vi "build token URI.vi"(8 "error in (no error)":errorcluster, 11 "Oauth2 in":refnum<class "Oauth2.lvclass">) -> (0 "error out":errorcluster, 1 "Headers":cluster{"header":string, "value":string}[](array[cluster]), 2 "Token Request URI":string, 3 "Oauth2":refnum<class "Oauth2.lvclass">)   [LabVIEW 2017, in "Oauth2.lvclass"]
uses:
  Oauth2.lvclass
  OAuthToken/OAuth2 Token Element -- enum.ctl
  Oauth2.lvclass/Oauth2.ctl
  <vilib>/LabVIEW Open Source Project/OpenURI/uri/URI.lvclass
  OAuthToken/OAuthAccessToken.lvclass
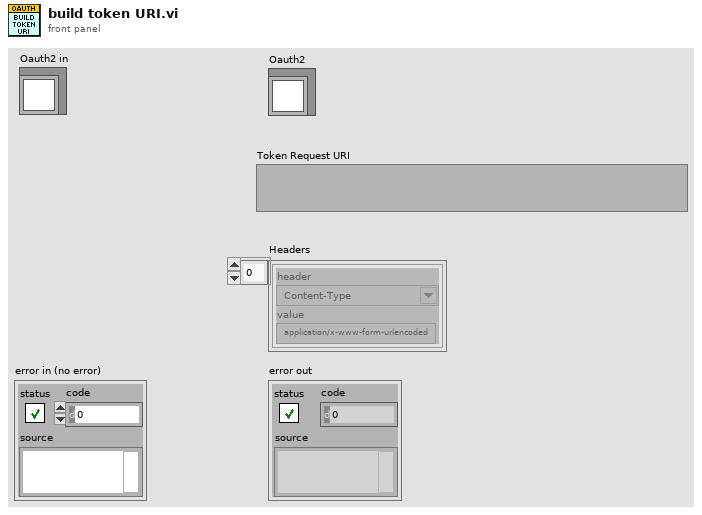
[diagram p1: front panel]
types:
  T1 = typedef "OAuthAccessToken.lvclass/OAuth2 Token Element -- enum.ctl" = enum16{"client_id", "client_secret", "response_type", "scope", "redirect_uri", "error", "error_description", "error_uri", "grant_type", "code", "access_token", "token_type", "expires_in", "username", "password", "refresh_token", "code_challenge", "code_challenge_method", "reverse_proxy_uri", "endpoint element", "access_type", "prompt", "id_token"}
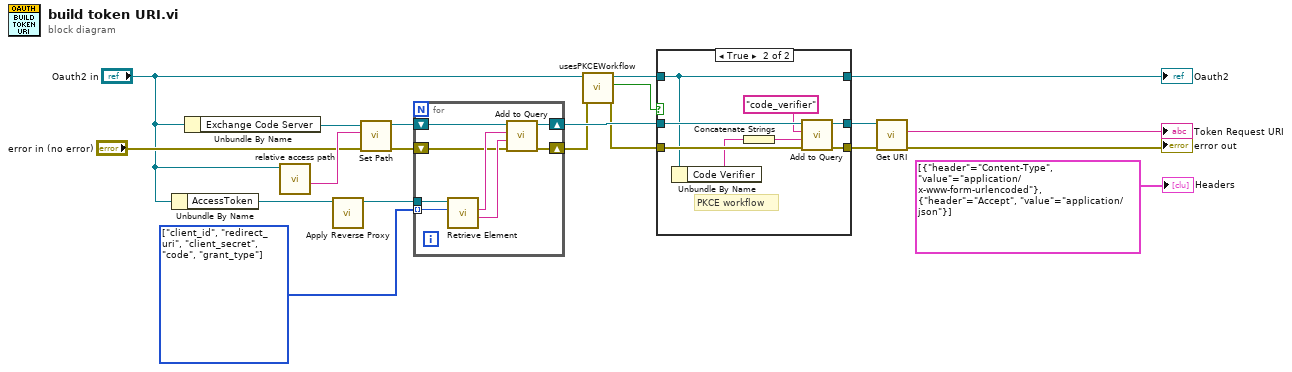
[diagram p0: block diagram]
diagram:
  w15 = T1[] [enum."client_id", enum."redirect_uri", enum."client_secret", enum."code", enum."grant_type"] items=["client_id", "client_secret", "response_type", "scope", "redirect_uri", "error", "error_description", "error_uri", "grant_type", "code", "access_token", "token_type", "expires_in", "username", "password", "refresh_token", "code_challenge", "code_challenge_method", "reverse_proxy_uri", "endpoint element", "access_type", "prompt", "id_token"]
  n1 = Unbundle By Name("Oauth2 in") -> ("AccessToken"=w3:refnum<class "OAuthAccessToken.lvclass">)
  n2 = Unbundle By Name("Oauth2 in") -> ("Exchange Code Server"=w17:refnum<class "URI.lvclass">)
  n3 = call-dynamic "relative access path.vi"("Oauth2 in"="Oauth2 in") -> ("Token Access Path"=w18:string)  [unwired: 9 in, 1 out]
  n4 = call "Apply Reverse Proxy.vi"("OAuthAccessToken in"=w3) -> ("OAuthAccessToken out"=w2:refnum<class "OAuthAccessToken.lvclass">)  [unwired: 9 in, 1 out]
  n5 = call <vilib>:"Set Path.vi"("error in (no error)"="error in (no error)", "path"=w18, "URI in"=w17) -> ("error out"=w13:errorcluster, "URI out"=w14:refnum<class "URI.lvclass">)  [unwired: 7 in]
  n6 = for {
    tunnel: w2 -> [w28]
    tunnel: w15 -> [w27] mode=indexing
    shift-right: [w25] -> w12
    shift-left: w14 -> [w26]
    shift-right: [w21] -> w8
    shift-left: w13 -> [w22]
    n7 = call "Retrieve Element.vi"("Token element"=w27, "OAuthAccessToken in"=w28) -> ("Value"=w23:string, "Key"=w24:string)  [unwired: 5 in, 3 out]
    n8 = call <vilib>:"Add to Query.vi"("error in (no error)"=w22, "value"=w23, "key"=w24, "URI in"=w26) -> ("error out"=w21:errorcluster, "URI out"=w25:refnum<class "URI.lvclass">)  [unwired: 6 in]
  }
  n9 = call "usesPKCEWorkflow.vi"("error in (no error)"=w8, "Oauth2 in"="Oauth2 in") -> ("error out"=w7:errorcluster, "PKCE?"=w1:bool, "Oauth2 out"=w6:refnum<class "Oauth2.lvclass">)  [unwired: 7 in]
  n10 = case shown="True" w1 {
    tunnel: w12 -> [w30 w39]
    tunnel: [w30 w38] -> w11
    tunnel: w7 -> [w31 w37]
    tunnel: [w31 w36] -> w10
    tunnel: w6 -> [w29 w34]
    tunnel: [w29 w34] -> w5
    frame False {
      # "code verifier for auth code\nonly, nor for access code\nFAILs with code_verifier and  \nLinkedIn"
    }
    frame True {
      # "PKCE workflow"
      n11 = Unbundle By Name(w34) -> ("Code Verifier"=w33:string)
      n12 = Concatenate Strings(w33) -> (w32:string)
      n13 = call <vilib>:"Add to Query.vi"("error in (no error)"=w37, "value"=w32, "key"="code_verifier", "URI in"=w39) -> ("error out"=w36:errorcluster, "URI out"=w38:refnum<class "URI.lvclass">)  [unwired: 6 in]
    }
  }
  "Oauth2" <- w5
  n14 = call <vilib>:"Get URI.vi"("error in (no error)"=w10, "URI in"=w11) -> ("error out"=→"error out":errorcluster, "URI String"=→"Token Request URI":string)  [unwired: 7 in, 1 out]
  "Headers" <- cluster{"header":string, "value":string}[] [{"header"="Content-Type", "value"="application/x-www-form-urlencoded"}, {"header"="Accept", "value"="application/json"}] ("Headers")
